vi "PID Autotuning Wizard.vi"(0 "states":T4(ring)=enum."Start", 1 "tuning completed?":bool, 5 "autotuning parameters":T2={"Controller Type"=0, "# of cycles to avg"=3, "Relay amplitude"=0.0, "Control design  "=0, "Noise level"=0.25} {"Noise level" format="%.2f"; "Control design" items=["Normal", "Fast", "Slow"]; "Relay amplitude" format="%.2f"; "Controller Type" items=["PID", "PI", "P"]}, 7 "Control Signals":T3 {"output" format="%.2f"; "setpoint" format="%.2f"; "process variable" format="%.2f"}, 9 "output range":cluster{"output high":dbl, "output low":dbl}={"output high"=100.0, "output low"=-100.0} {"output low" format="%.2f"; "output high" format="%.2f"}, 11 "dt (s)":dbl=1.0 format="%.3f", 12 "new PID parameters input":T1 {"Td (min)" format="%.4f"; "Ti (min)" format="%.4f"; "Kc" format="%.4f"}) -> (4 "state out":T4(ring)=enum."Start", 6 "autotuning parameters out":T2={"Controller Type"=0, "# of cycles to avg"=3, "Relay amplitude"=0.0, "Control design  "=0, "Noise level"=0.25} {"Noise level" format="%.2f"; "Control design" items=["Normal", "Fast", "Slow"]; "Relay amplitude" format="%.2f"; "Controller Type" items=["PID", "PI", "P"]}, 10 "complete?":bool, 14 "yes/no out":bool, 15 "new PID parameters out":T1 {"Td (min)" format="%.4f"; "Ti (min)" format="%.4f"; "Kc" format="%.4f"})   [LabVIEW 2020, in "NI_PID_autopid.lvlib"]
doc: "The Current noise level estimate parameter is used during the setpoint relay experiment. At this step, the process is still under normal PID control.\n\nYou can enter a value directly if you know the approximate magnitude of the noise in the measurement of the process variable. This value corresponds to the mean square error of the process variable at steady state. Alternatively, the Autotuning Wizard can make a measure of this value for you. Select Re-estimate to choose this option.\n\nThe noise level estimate is used during the setpoint relay experiment to prevent noise on the process variable from triggering the relay. The autotuning algorithm uses this noise level estimate as a hysteresis for the relay action."
uses:
  <vilib>/addons/control/pid/NI_PID_autopid.lvlib
panel:
  in  "Warning":string="Warning: Ti is zero!"
  out "Previous PID Parameters":T1 {"Td (min)" format="%#.6g"; "Ti (min)" format="%#.6g"; "Kc" format="%#.6g"}
  in  "OK":bool
  out "yes/no":bool
  in  "Accept current value":bool
  in  "Re-estimate noise level":bool
  in  "current parameters":T5={"Controller type"=0, "Cycles to average"=3, "Relay amplitude"=0.0, "Control design"=0, "Noise level %"=0.25} {"Noise level %" format="%.2f"; "Control design" items=["Normal", "Fast", "Slow"]; "Relay amplitude" min=0.0 format="%#.6g"; "Cycles to average" min=1; "Controller type" items=["PID", "PI", "P"]}
  in  "Cancel":bool
  in  "Next":bool
  in  "Back":bool
  out "VI name":string
  in  "Current noise level estimate":dbl format="%#.6g"
  out "New PID Parameters":T1 {"Td (min)" format="%#.6g"; "Ti (min)" format="%#.6g"; "Kc" format="%#.6g"}
  out "Process Monitor":T6(graph)={"PV%"=28.332617282818244, "setpoint (%)"=28.30188679245283, "output (%)"=13.51595979484235}
  out "Instructions":string
  in  "no":bool
  in  "yes":bool
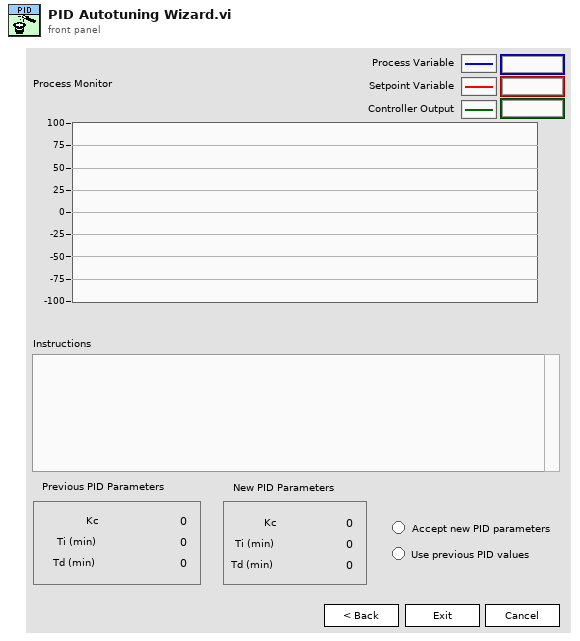
[diagram p1: front panel]
types:
  T1 = cluster{"Kc":dbl, "Ti (min)":dbl, "Td (min)":dbl}
  T2 = cluster{"Controller Type":u16, "# of cycles to avg":i32, "Relay amplitude":dbl, "Control design  ":u16, "Noise level":dbl}
  T3 = cluster{"process variable":dbl, "setpoint":dbl, "output":dbl}
  T4 = enum16{"Normal", "Start", "Check params", "Check noise", "Start noise est.", "Re-estimate noise", "Begin autotune", "Autotuning", "New parameters", ""}
  T5 = cluster{"Controller type":u16, "Cycles to average":i32, "Relay amplitude":dbl, "Control design":u16, "Noise level %":dbl}
  T6 = cluster{"PV%":dbl, "setpoint (%)":dbl, "output (%)":dbl}
  T7 = cluster{"PV%":dbl, "setpoint (%)":dbl, "output (%)":dbl}[]
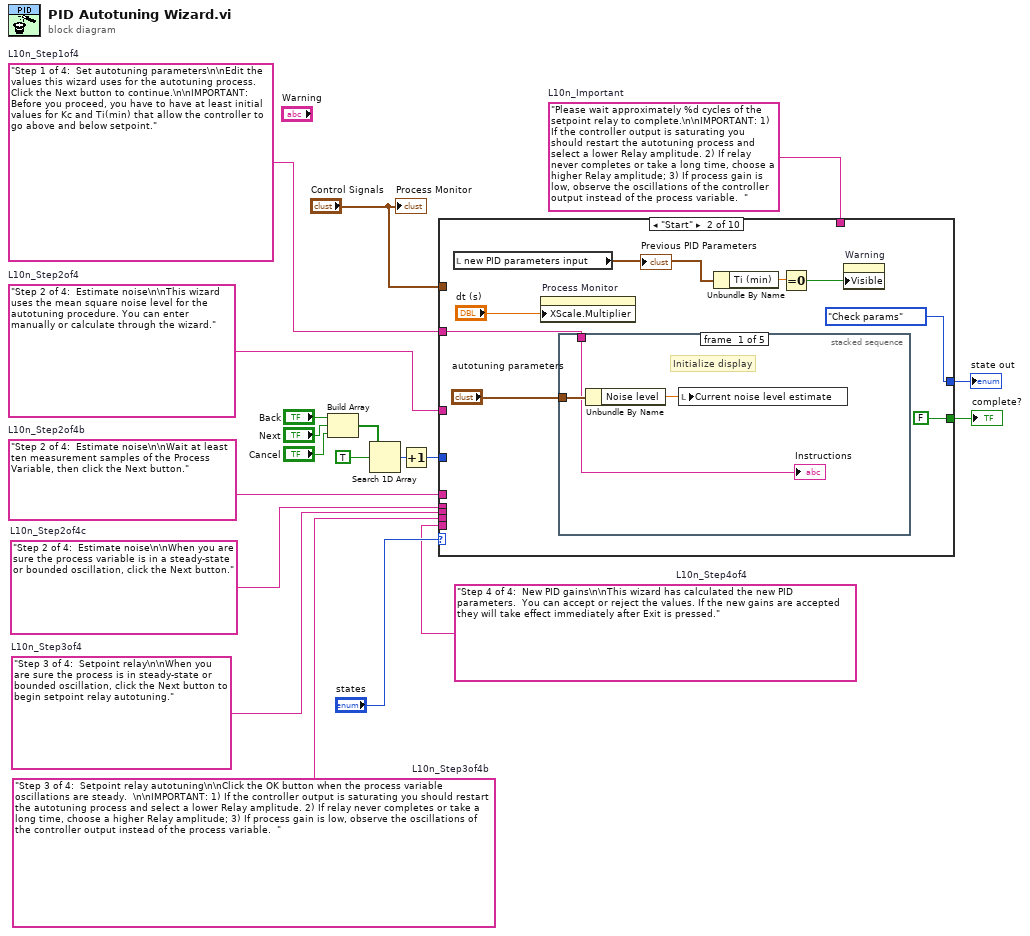
[diagram p0: block diagram]
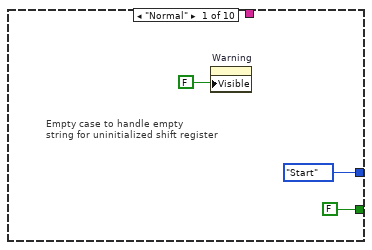
[diagram p2: hidden frame]
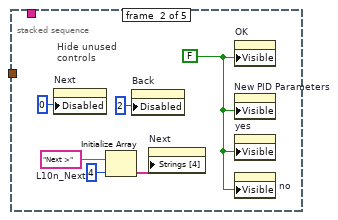
[diagram p3: hidden frame]
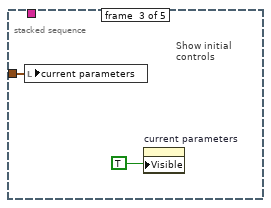
[diagram p4: hidden frame]
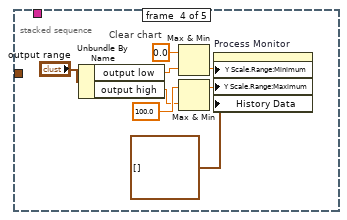
[diagram p5: hidden frame]
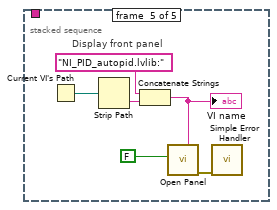
[diagram p6: hidden frame]
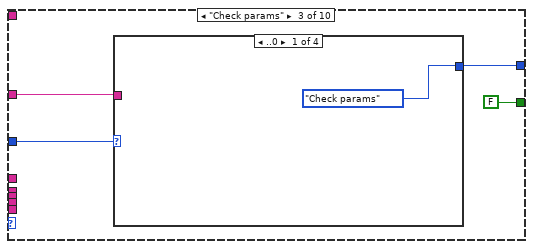
[diagram p7: hidden frame]
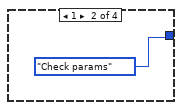
[diagram p8: hidden frame]
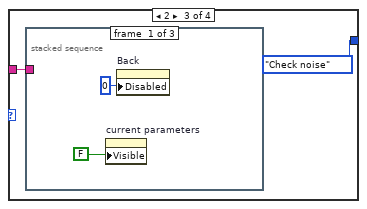
[diagram p9: hidden frame]
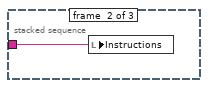
[diagram p10: hidden frame]
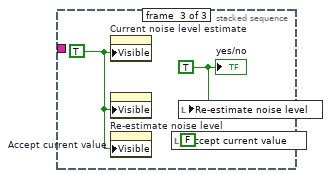
[diagram p11: hidden frame]
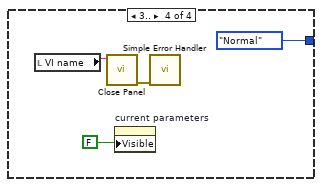
[diagram p12: hidden frame]
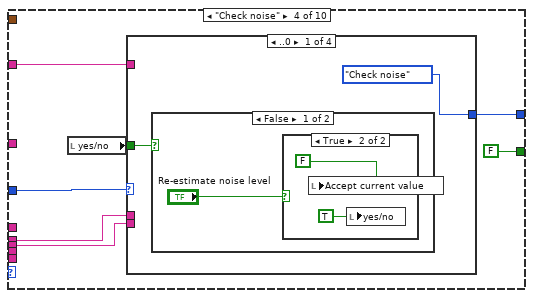
[diagram p13: hidden frame]
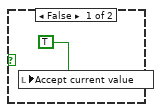
[diagram p14: hidden frame]
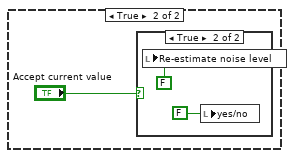
[diagram p15: hidden frame]
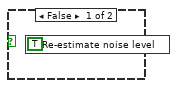
[diagram p16: hidden frame]
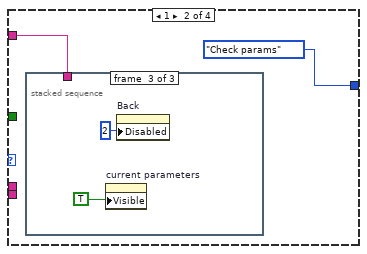
[diagram p17: hidden frame]
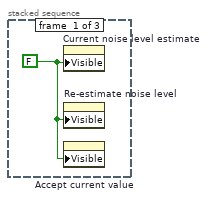
[diagram p18: hidden frame]
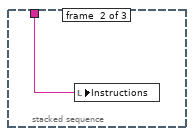
[diagram p19: hidden frame]
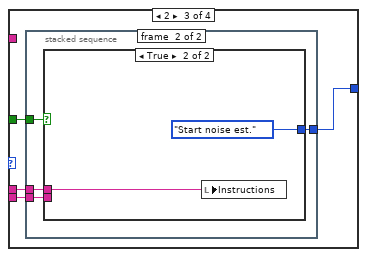
[diagram p20: hidden frame]
diagram:
  w1 = "Please wait approximately %d cycles of the setpoint relay to complete.\n\nIMPORTANT: 1) If the controller output is saturating you should restart the autotuning process and select a lower Relay amplitude. 2) If relay never completes or take a long time, choose a higher Relay amplitude; 3) If process gain is low, observe the oscillations of the controller output instead of the process variable.  "  # L10n_Important
  w2 = "Step 4 of 4:  New PID gains\n\nThis wizard has calculated the new PID parameters.  You can accept or reject the values. If the new gains are accepted they will take effect immediately after Exit is pressed."  # L10n_Step4of4
  w3 = "Step 3 of 4:  Setpoint relay autotuning\n\nClick the OK button when the process variable oscillations are steady.  \n\nIMPORTANT: 1) If the controller output is saturating you should restart the autotuning process and select a lower Relay amplitude. 2) If relay never completes or take a long time, choose a higher Relay amplitude; 3) If process gain is low, observe the oscillations of the controller output instead of the process variable.  "  # L10n_Step3of4b
  w4 = "Step 3 of 4:  Setpoint relay\n\nWhen you are sure the process is in steady-state or bounded oscillation, click the Next button to begin setpoint relay autotuning."  # L10n_Step3of4
  w5 = "Step 2 of 4:  Estimate noise\n\nWhen you are sure the process variable is in a steady-state or bounded oscillation, click the Next button."  # L10n_Step2of4c
  w6 = "Step 2 of 4:  Estimate noise\n\nWait at least ten measurement samples of the Process Variable, then click the Next button."  # L10n_Step2of4b
  w7 = "Step 1 of 4:  Set autotuning parameters\n\nEdit the values this wizard uses for the autotuning process. Click the Next button to continue.\n\nIMPORTANT: Before you proceed, you have to have at least initial values for Kc and Ti(min) that allow the controller to go above and below setpoint."  # L10n_Step1of4
  w8 = "Step 2 of 4:  Estimate noise\n\nThis wizard uses the mean square noise level for the autotuning procedure. You can enter manually or calculate through the wizard."  # L10n_Step2of4
  n1 = Build Array("Back", "Next", "Cancel") -> (w19:bool[])
  n2 = Search 1D Array(1D array=w19, element=TRUE) -> (index of element=w18:i32)  [unwired: 1 out]
  n3 = Increment(x=w18) -> (x+1=w13:i32)
  n4 = case shown="\"Start\"" "states" {
    tunnel: [T4."Start" ("states") T4."Check params" ("states") w57 w78 w119 w137 w159 w181 w219 T4."Start" ("states")] -> w12
    tunnel: [FALSE FALSE FALSE FALSE FALSE FALSE FALSE FALSE w218 FALSE] -> w10
    tunnel: w13 -> [_ _ w58 w79 w120 w138 w160 w182 w220 _]
    tunnel: "Control Signals" -> [_ _ _ _ _ w136 _ _ _ _]
    tunnel: w8 -> [_ _ w56 _ w118 w134 w157 w178 _ _]
    tunnel: w7 -> [_ w27 _ w76 _ _ _ _ _ _]
    tunnel: w6 -> [_ _ _ _ w117 _ _ _ _ _]
    tunnel: w5 -> [_ _ _ w75 _ w133 _ _ _ _]
    tunnel: w4 -> [_ _ _ w74 _ _ _ _ w217 _]
    tunnel: w3 -> [_ _ _ _ _ _ w156 _ _ _]
    tunnel: w2 -> [_ _ _ _ _ _ _ w177 _ _]
    tunnel: w1 -> [_ _ _ _ _ _ _ w176 _ _]
    frame "Normal" {
      # "Empty case to handle empty\nstring for uninitialized shift register"
      n5 = property on="Warning" class="Str"("Visible"=FALSE) -> ()  [unwired: 2 in, 2 out]
    }
    frame "Start" {
      n6 = local read "new PID parameters input"() -> (w25:T1)
      "Previous PID Parameters" <- w25
      n7 = property on="Process Monitor" class="WFChart (strict)"("XScale.Multiplier"="dt (s)") -> ()  [unwired: 2 in, 2 out]
      n8 = stacked-sequence {
        tunnel: "autotuning parameters" -> [w33 _ w40 _ _]
        tunnel: w27 -> [w31 _ _ _ _]
        frame #0 {
          # "Initialize display"
          n9 = Unbundle By Name(w33) -> ("Noise level"=w32:dbl)
          n10 = local write "Current noise level estimate"(w32) -> ()
          "Instructions" <- w31
        }
        frame #1 {
          w35 = "Next >"  # L10n_Next
          w39 = FALSE ("Visible")
          # "Hide unused\ncontrols"
          n11 = property on="Next" class="Bool"("Disabled"=u8 0) -> ()  [unwired: 2 in, 2 out]
          n12 = Initialize Array(w35, 4) -> (w34:string[])
          n13 = property on="Back" class="Bool"("Disabled"=u8 2) -> ()  [unwired: 2 in, 2 out]
          n14 = property on="Next" class="Bool"("Strings [4]"=w34) -> ()  [unwired: 2 in, 2 out]
          n15 = property on="OK" class="Bool (strict)"("Visible"=w39) -> ()  [unwired: 2 in, 2 out]
          n16 = property on="New PID Parameters" class="Clust (strict)"("Visible"=w39) -> ()  [unwired: 2 in, 2 out]
          n17 = property on="yes" class="Bool (strict)"("Visible"=w39) -> ()  [unwired: 2 in, 2 out]
          n18 = property on="no" class="Bool (strict)"("Visible"=w39) -> ()  [unwired: 2 in, 2 out]
        }
        frame #2 {
          # "Show initial\ncontrols"
          n19 = local write "current parameters"(w40) -> ()
          n20 = property on="current parameters" class="Clust (strict)"("Visible"=TRUE) -> ()  [unwired: 2 in, 2 out]
        }
        frame #3 {
          # "Clear chart"
          n21 = Unbundle By Name("output range") -> ("output low"=w43:dbl, "output high"=w42:dbl)
          n22 = Max & Min(x=0.0, y=w43) -> (min(x,y)=w49:dbl)  [unwired: 1 out]
          n23 = Max & Min(x=100.0, y=w42) -> (max(x,y)=w48:dbl)  [unwired: 1 out]
          n24 = property on="Process Monitor" class="WFChart (strict)"("Y Scale.Range:Minimum"=w49, "Y Scale.Range:Maximum"=w48, "History Data"=T7 []) -> ()  [unwired: 2 in, 2 out]
        }
        frame #4 {
          # "Display front panel"
          n25 = Current VI's Path() -> (path=w54:path)
          n26 = Strip Path(path=w54) -> (name=w53:string)  [unwired: 1 out]
          n27 = Concatenate Strings("NI_PID_autopid.lvlib:" ("string"), w53) -> (w51:string)
          "VI name" <- w51
          n28 = call <vilib>:"Open Panel.vi"("use VI Setup settings? (T)"=FALSE, "VI name"=w51) -> ("error out"=w55:errorcluster)  [unwired: 1 in, 8 out]
          n29 = call <vilib>:"Simple Error Handler.vi"("error in (no error)"=w55) -> ()  [unwired: 1 in, 8 out]
        }
      }
      n30 = Unbundle By Name(w25) -> ("Ti (min)"=w24:dbl)
      n31 = Equal To 0?(x=w24) -> (x = 0?=w23:bool)
      n32 = property on="Warning" class="Str"("Visible"=w23) -> ()  [unwired: 2 in, 2 out]
    }
    frame "Check params" {
      n33 = case shown="..0" w58 {
        tunnel: [T4."Check params" ("states") T4."Check params" ("states") T4."Check noise" ("states") T4."Normal" ("states")] -> w57
        tunnel: w56 -> [_ _ w62 _]
        frame ..0 {
        }
        frame 1 {
        }
        frame 2 {
          n34 = stacked-sequence {
            tunnel: w62 -> [_ w66 _]
            frame #0 {
              n35 = property on="current parameters" class="Clust (strict)"("Visible"=FALSE) -> ()  [unwired: 2 in, 2 out]
              n36 = property on="Back" class="Bool"("Disabled"=u8 0) -> ()  [unwired: 2 in, 2 out]
            }
            frame #1 {
              n37 = local write "Instructions"(w66) -> ()
            }
            frame #2 {
              w68 = TRUE ("yes/no")
              w69 = TRUE ("Visible")
              n38 = property on="Current noise level estimate" class="DigNum (strict)"("Visible"=w69) -> ()  [unwired: 2 in, 2 out]
              n39 = property on="Re-estimate noise level" class="Bool (strict)"("Visible"=w69) -> ()  [unwired: 2 in, 2 out]
              n40 = property on="Accept current value" class="Bool (strict)"("Visible"=w69) -> ()  [unwired: 2 in, 2 out]
              n41 = local write "Accept current value"(FALSE ("Accept")) -> ()
              n42 = local write "Re-estimate noise level"(w68) -> ()
              "yes/no" <- w68
            }
          }
        }
        frame 3.. {
          n43 = local read "VI name"() -> (w71:string)
          n44 = call <vilib>:"Close Panel.vi"("VI name"=w71) -> ("error out"=w72:errorcluster)  [unwired: 1 in, 9 out]
          n45 = property on="current parameters" class="Clust (strict)"("Visible"=FALSE) -> ()  [unwired: 2 in, 2 out]
          n46 = call <vilib>:"Simple Error Handler.vi"("error in (no error)"=w72) -> ()  [unwired: 1 in, 8 out]
        }
      }
    }
    frame "Check noise" {
      n47 = local read "yes/no"() -> (w77:bool)
      n48 = case shown="..0" w79 {
        tunnel: [T4."Check noise" ("states") T4."Check params" ("states") w99 T4."Normal" ("states")] -> w78
        tunnel: w77 -> [w82 _ w100 _]
        tunnel: w76 -> [_ w91 _ _]
        tunnel: w75 -> [_ _ w98 _]
        tunnel: w74 -> [_ _ w97 _]
        frame ..0 {
          n49 = case shown="False" w82 {
            frame False {
              n50 = case shown="True" "Re-estimate noise level" {
                frame False {
                  n51 = local write "Accept current value"(TRUE ("Accept")) -> ()
                }
                frame True {
                  n52 = local write "Accept current value"(FALSE ("Re-estimate")) -> ()
                  n53 = local write "yes/no"(TRUE ("yes/no")) -> ()
                }
              }
            }
            frame True {
              n54 = case shown="True" "Accept current value" {
                frame False {
                  n55 = local write "Re-estimate noise level"(TRUE ("Re-estimate")) -> ()
                }
                frame True {
                  n56 = local write "Re-estimate noise level"(FALSE ("Re-estimate")) -> ()
                  n57 = local write "yes/no"(FALSE ("yes/no")) -> ()
                }
              }
            }
          }
        }
        frame 1 {
          n58 = stacked-sequence {
            tunnel: w91 -> [_ w94 _]
            frame #0 {
              w93 = FALSE ("Visible")
              n59 = property on="Current noise level estimate" class="DigNum (strict)"("Visible"=w93) -> ()  [unwired: 2 in, 2 out]
              n60 = property on="Re-estimate noise level" class="Bool (strict)"("Visible"=w93) -> ()  [unwired: 2 in, 2 out]
              n61 = property on="Accept current value" class="Bool (strict)"("Visible"=w93) -> ()  [unwired: 2 in, 2 out]
            }
            frame #1 {
              n62 = local write "Instructions"(w94) -> ()
            }
            frame #2 {
              n63 = property on="current parameters" class="Clust (strict)"("Visible"=TRUE) -> ()  [unwired: 2 in, 2 out]
              n64 = property on="Back" class="Bool"("Disabled"=u8 2) -> ()  [unwired: 2 in, 2 out]
            }
          }
        }
        frame 2 {
          n65 = stacked-sequence {
            tunnel: w100 -> [_ w105]
            tunnel: [_ w104] -> w99
            tunnel: w98 -> [_ w103]
            tunnel: w97 -> [_ w102]
            frame #0 {
              w101 = FALSE ("Visible")
              n66 = property on="Current noise level estimate" class="DigNum (strict)"("Visible"=w101) -> ()  [unwired: 2 in, 2 out]
              n67 = property on="Re-estimate noise level" class="Bool (strict)"("Visible"=w101) -> ()  [unwired: 2 in, 2 out]
              n68 = property on="Accept current value" class="Bool (strict)"("Visible"=w101) -> ()  [unwired: 2 in, 2 out]
            }
            frame #1 {
              n69 = case shown="True" w105 {
                tunnel: [T4."Begin autotune" ("states") T4."Start noise est." ("states")] -> w104
                tunnel: w103 -> [_ w111]
                tunnel: w102 -> [w106 _]
                frame False {
                  n70 = local read "current parameters"() -> (w108:T5)
                  n71 = Bundle By Name(cluster=w108, "Noise level %"="Current noise level estimate") -> (w110:T5)
                  n72 = local write "Instructions"(w106) -> ()
                  n73 = local write "current parameters"(w110) -> ()
                }
                frame True {
                  n74 = local write "Instructions"(w111) -> ()
                }
              }
            }
          }
        }
        frame 3.. {
          w114 = FALSE ("Visible")
          n75 = property on="Current noise level estimate" class="DigNum (strict)"("Visible"=w114) -> ()  [unwired: 2 in, 2 out]
          n76 = property on="Re-estimate noise level" class="Bool (strict)"("Visible"=w114) -> ()  [unwired: 2 in, 2 out]
          n77 = property on="Accept current value" class="Bool (strict)"("Visible"=w114) -> ()  [unwired: 2 in, 2 out]
          n78 = local read "VI name"() -> (w115:string)
          n79 = call <vilib>:"Close Panel.vi"("VI name"=w115) -> ("error out"=w116:errorcluster)  [unwired: 1 in, 9 out]
          n80 = call <vilib>:"Simple Error Handler.vi"("error in (no error)"=w116) -> ()  [unwired: 1 in, 8 out]
        }
      }
    }
    frame "Start noise est." {
      n81 = case shown="3.." w120 {
        tunnel: [T4."Start noise est." ("states") T4."Check noise" ("states") T4."Re-estimate noise" ("states") T4."Normal" ("states")] -> w119
        tunnel: w118 -> [_ w123 _ _]
        tunnel: w117 -> [_ _ w127 _]
        frame ..0 {
        }
        frame 1 {
          n82 = stacked-sequence {
            tunnel: w123 -> [_ w126]
            frame #0 {
              w125 = TRUE ("Visible")
              n83 = property on="Current noise level estimate" class="DigNum (strict)"("Visible"=w125) -> ()  [unwired: 2 in, 2 out]
              n84 = property on="Re-estimate noise level" class="Bool (strict)"("Visible"=w125) -> ()  [unwired: 2 in, 2 out]
              n85 = property on="Accept current value" class="Bool (strict)"("Visible"=w125) -> ()  [unwired: 2 in, 2 out]
            }
            frame #1 {
              n86 = local write "Instructions"(w126) -> ()
            }
          }
        }
        frame 2 {
          n87 = call <vilib>:"PID MeaNoise.vi"("OK"=FALSE) -> ()  [unwired: 1 in, 2 out]
          n88 = local write "Instructions"(w127) -> ()
        }
        frame 3.. {
          n89 = local read "VI name"() -> (w131:string)
          n90 = call <vilib>:"Close Panel.vi"("VI name"=w131) -> ("error out"=w132:errorcluster)  [unwired: 1 in, 9 out]
          n91 = call <vilib>:"Simple Error Handler.vi"("error in (no error)"=w132) -> ()  [unwired: 1 in, 8 out]
        }
      }
    }
    frame "Re-estimate noise" {
      n92 = Unbundle By Name(w136) -> ("process variable"=w135:dbl)
      n93 = case shown="..0" w138 {
        tunnel: [T4."Re-estimate noise" ("states") T4."Start noise est." ("states") T4."Check noise" ("states") T4."Normal" ("states")] -> w137
        tunnel: w135 -> [w141 _ _ _]
        tunnel: w134 -> [_ _ w145 _]
        tunnel: w133 -> [_ w143 _ _]
        frame ..0 {
          n94 = call <vilib>:"PID MeaNoise.vi"("OK"=TRUE, "PV %"=w141) -> ()  [unwired: 2 out]
        }
        frame 1 {
          n95 = local write "Instructions"(w143) -> ()
        }
        frame 2 {
          n96 = stacked-sequence {
            tunnel: w145 -> [_ _ w152]
            frame #0 {
              n97 = call <vilib>:"PID MeaNoise.vi"("OK"=FALSE) -> ("Noise"=w147:dbl)  [unwired: 1 in, 1 out]
              n98 = local write "Current noise level estimate"(w147) -> ()
            }
            frame #1 {
              w150 = FALSE ("yes/no")
              w151 = TRUE ("Visible")
              n99 = property on="Current noise level estimate" class="DigNum (strict)"("Visible"=w151) -> ()  [unwired: 2 in, 2 out]
              n100 = property on="Re-estimate noise level" class="Bool (strict)"("Visible"=w151) -> ()  [unwired: 2 in, 2 out]
              n101 = property on="Accept current value" class="Bool (strict)"("Visible"=w151) -> ()  [unwired: 2 in, 2 out]
              n102 = local write "Re-estimate noise level"(w150) -> ()
              n103 = local write "Accept current value"(TRUE ("Accept")) -> ()
              n104 = local write "yes/no"(w150) -> ()
            }
            frame #2 {
              n105 = local write "Instructions"(w152) -> ()
            }
          }
        }
        frame 3.. {
          n106 = local read "VI name"() -> (w154:string)
          n107 = call <vilib>:"Close Panel.vi"("VI name"=w154) -> ("error out"=w155:errorcluster)  [unwired: 1 in, 9 out]
          n108 = call <vilib>:"Simple Error Handler.vi"("error in (no error)"=w155) -> ()  [unwired: 1 in, 8 out]
        }
      }
    }
    frame "Begin autotune" {
      n109 = local read "current parameters"() -> (→"autotuning parameters out":T5)
      n110 = case shown="1" w160 {
        tunnel: [T4."Begin autotune" ("states") T4."Check noise" ("states") T4."Autotuning" ("states") T4."Normal" ("states")] -> w159
        tunnel: w157 -> [_ w163 _ _]
        tunnel: w156 -> [_ _ w167 _]
        frame ..0 {
        }
        frame 1 {
          n111 = stacked-sequence {
            tunnel: w163 -> [_ w166]
            frame #0 {
              w165 = TRUE ("Visible")
              n112 = property on="Current noise level estimate" class="DigNum (strict)"("Visible"=w165) -> ()  [unwired: 2 in, 2 out]
              n113 = property on="Re-estimate noise level" class="Bool (strict)"("Visible"=w165) -> ()  [unwired: 2 in, 2 out]
              n114 = property on="Accept current value" class="Bool (strict)"("Visible"=w165) -> ()  [unwired: 2 in, 2 out]
            }
            frame #1 {
              n115 = local write "Instructions"(w166) -> ()
            }
          }
        }
        frame 2 {
          n116 = property on="OK" class="Bool (strict)"("Visible"=TRUE, "Disabled"=u8 0) -> ()  [unwired: 2 in, 2 out]
          n117 = property on="Next" class="Bool"("Disabled"=u8 2) -> ()  [unwired: 2 in, 2 out]
          n118 = local write "Instructions"(w167) -> ()
          n119 = local write "OK"(FALSE ("OK")) -> ()
        }
        frame 3.. {
          n120 = local read "VI name"() -> (w174:string)
          n121 = call <vilib>:"Close Panel.vi"("VI name"=w174) -> ("error out"=w175:errorcluster)  [unwired: 1 in, 9 out]
          n122 = call <vilib>:"Simple Error Handler.vi"("error in (no error)"=w175) -> ()  [unwired: 1 in, 8 out]
        }
      }
    }
    frame "Autotuning" {
      n123 = case shown="3.." w182 {
        tunnel: [w191 T4."Check noise" ("states") T4."Autotuning" ("states") T4."Normal" ("states")] -> w181
        tunnel: w178 -> [_ w207 _ _]
        tunnel: w177 -> [w189 _ _ _]
        frame ..0 {
          n124 = case shown="False" "tuning completed?" {
            tunnel: [T4."Autotuning" ("states") w194] -> w191
            tunnel: w189 -> [_ w193]
            frame False {
            }
            frame True {
              n125 = stacked-sequence {
                tunnel: [_ _ T4."New parameters" ("states") _] -> w194
                tunnel: w193 -> [_ _ w201 _]
                frame #0 {
                  n126 = local write "yes/no"(TRUE ("yes/no")) -> ()
                  n127 = local write "OK"(FALSE ("OK")) -> ()
                  n128 = property on="OK" class="Bool (strict)"("Visible"=FALSE, "Disabled"=u8 0) -> ()  [unwired: 2 in, 2 out]
                  "New PID Parameters" <- "new PID parameters input"
                }
                frame #1 {
                  w200 = TRUE ("Visible")
                  n129 = property on="New PID Parameters" class="Clust (strict)"("Visible"=w200) -> ()  [unwired: 2 in, 2 out]
                  n130 = property on="yes" class="Bool (strict)"("Visible"=w200) -> ()  [unwired: 2 in, 2 out]
                  n131 = property on="no" class="Bool (strict)"("Visible"=w200) -> ()  [unwired: 2 in, 2 out]
                }
                frame #2 {
                  n132 = local write "Instructions"(w201) -> ()
                }
                frame #3 {
                  w205 = "Exit"  # L10n_Exit
                  n133 = Initialize Array(w205, 4) -> (w204:string[])
                  n134 = property on="Next" class="Bool"("Strings [4]"=w204) -> ()  [unwired: 2 in, 2 out]
                  n135 = property on="Next" class="Bool"("Disabled"=u8 0) -> ()  [unwired: 2 in, 2 out]
                }
              }
            }
          }
        }
        frame 1 {
          n136 = stacked-sequence {
            tunnel: w207 -> [_ w212]
            frame #0 {
              w211 = TRUE ("Visible")
              n137 = property on="Current noise level estimate" class="DigNum (strict)"("Visible"=w211) -> ()  [unwired: 2 in, 2 out]
              n138 = property on="Re-estimate noise level" class="Bool (strict)"("Visible"=w211) -> ()  [unwired: 2 in, 2 out]
              n139 = property on="Accept current value" class="Bool (strict)"("Visible"=w211) -> ()  [unwired: 2 in, 2 out]
              n140 = property on="Next" class="Bool"("Disabled"=u8 0) -> ()  [unwired: 2 in, 2 out]
              n141 = property on="OK" class="Bool (strict)"("Visible"=FALSE) -> ()  [unwired: 2 in, 2 out]
            }
            frame #1 {
              n142 = local write "Instructions"(w212) -> ()
            }
          }
        }
        frame 2 {
        }
        frame 3.. {
          n143 = local read "VI name"() -> (w215:string)
          n144 = call <vilib>:"Close Panel.vi"("VI name"=w215) -> ("error out"=w216:errorcluster)  [unwired: 1 in, 9 out]
          n145 = call <vilib>:"Simple Error Handler.vi"("error in (no error)"=w216) -> ()  [unwired: 1 in, 8 out]
        }
      }
      n146 = local write "yes/no"("OK") -> ()
      n147 = case shown="True" "OK" {
        tunnel: "current parameters" -> [_ w188]
        tunnel: w176 -> [_ w184]
        frame False {
        }
        frame True {
          n148 = Unbundle By Name(w188) -> ("Cycles to average"=w186:i32)
          n149 = property on="OK" class="Bool (strict)"("Disabled"=u8 2) -> ()  [unwired: 2 in, 2 out]
          n150 = Format Into String(format string=w184, w186) -> (resulting string=w185:string)  [unwired: 2 in, 1 out]
          n151 = local write "Instructions"(w185) -> ()
        }
      }
      "yes/no out" <- "OK"
    }
    frame "New parameters" {
      n152 = case shown="3.." w220 {
        tunnel: [T4."New parameters" ("states") T4."Begin autotune" ("states") T4."Normal" ("states") T4."Normal" ("states")] -> w219
        tunnel: [FALSE FALSE TRUE FALSE] -> w218
        tunnel: w217 -> [_ w232 _ _]
        frame ..0 {
          n153 = local read "yes/no"() -> (w222:bool)
          n154 = case shown="True" w222 {
            frame False {
              n155 = case shown="True" "yes" {
                frame False {
                  n156 = local write "no"(TRUE ("Accept")) -> ()
                }
                frame True {
                  n157 = local write "yes/no"(TRUE ("yes/no")) -> ()
                  n158 = local write "no"(FALSE ("Re-estimate")) -> ()
                }
              }
            }
            frame True {
              n159 = case shown="True" "no" {
                frame False {
                  n160 = local write "yes"(TRUE ("Re-estimate")) -> ()
                }
                frame True {
                  n161 = local write "yes/no"(FALSE ("yes/no")) -> ()
                  n162 = local write "yes"(FALSE ("Re-estimate")) -> ()
                }
              }
            }
          }
        }
        frame 1 {
          n163 = stacked-sequence {
            tunnel: w232 -> [_ w236 _]
            frame #0 {
              w235 = FALSE ("Visible")
              n164 = property on="New PID Parameters" class="Clust (strict)"("Visible"=w235) -> ()  [unwired: 2 in, 2 out]
              n165 = property on="yes" class="Bool (strict)"("Visible"=w235) -> ()  [unwired: 2 in, 2 out]
              n166 = property on="no" class="Bool (strict)"("Visible"=w235) -> ()  [unwired: 2 in, 2 out]
            }
            frame #1 {
              n167 = local write "Instructions"(w236) -> ()
            }
            frame #2 {
              w238 = "Next >"  # L10n_Next
              n168 = Initialize Array(w238, 4) -> (w237:string[])
              n169 = property on="Next" class="Bool"("Strings [4]"=w237) -> ()  [unwired: 2 in, 2 out]
            }
          }
        }
        frame 2 {
          n170 = local read "New PID Parameters"() -> (→"new PID parameters out":T1)
          n171 = local read "yes/no"() -> (w242:bool)
          n172 = local write "yes/no out"(w242) -> ()
          n173 = local read "VI name"() -> (w243:string)
          n174 = call <vilib>:"Close Panel.vi"("VI name"=w243) -> ("error out"=w244:errorcluster)  [unwired: 1 in, 9 out]
          n175 = call <vilib>:"Simple Error Handler.vi"("error in (no error)"=w244) -> ()  [unwired: 1 in, 8 out]
        }
        frame 3.. {
          n176 = local read "VI name"() -> (w248:string)
          n177 = call <vilib>:"Close Panel.vi"("VI name"=w248) -> ("error out"=w249:errorcluster)  [unwired: 1 in, 9 out]
          n178 = call <vilib>:"Simple Error Handler.vi"("error in (no error)"=w249) -> ()  [unwired: 1 in, 8 out]
        }
      }
    }
    frame "" {
      # "Empty case to handle empty\nstring for uninitialized shift register"
    }
  }
  "state out" <- w12
  "complete?" <- w10
  "Process Monitor" <- "Control Signals"
